vi "Read Flow Cal.vi"(8 "error in":errorcluster) -> (0 "error out":errorcluster, 2 "FM1-60":dbl[][](array[numeric]), 3 "FM1-20":dbl[][](array[numeric]))   [LabVIEW 2018]
uses:
  <vilib>/Utility/file.llb/Read Delimited Spreadsheet (DBL).vi
panel:
  # "GPM    HZ"
  # "GPM"
  # "HZ"
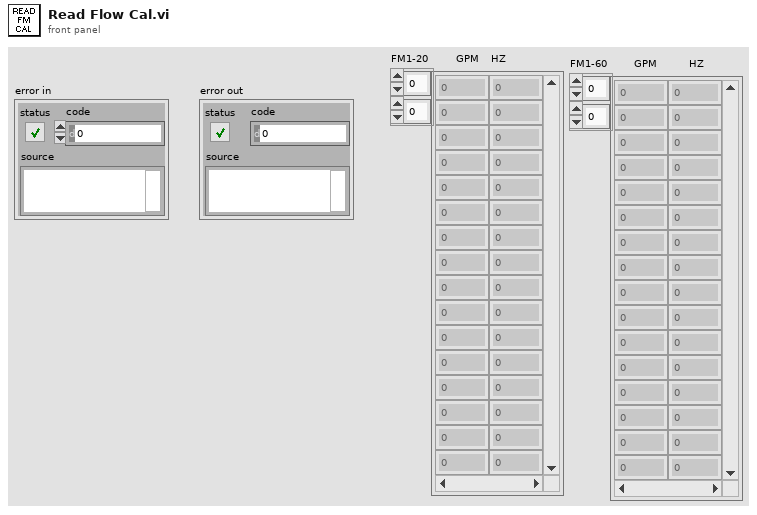
[diagram p1: front panel]
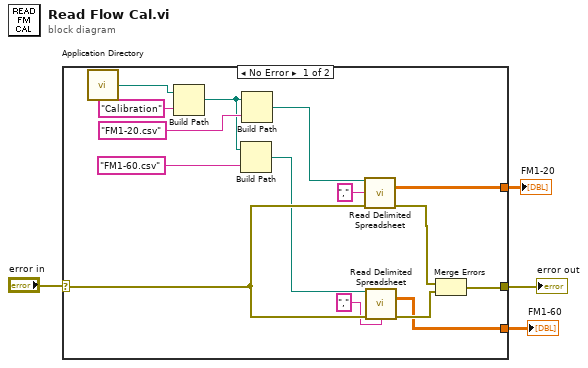
[diagram p0: block diagram]
diagram:
  n1 = case shown="No Error" "error in" {
    selector: "error in" -> [w19 w20]
    tunnel: [w12 w20] -> w3
    tunnel: [w6 _] -> w2
    tunnel: [w5 _] -> w1
    frame No Error {
      n2 = call <vilib>:"Application Directory.vi"() -> ("Application Directory"=w9:path)
      n3 = Build Path(base path=w9, name or relative path="Calibration") -> (appended path=w7:path)
      n4 = Build Path(base path=w7, name or relative path="FM1-60.csv") -> (appended path=w15:path)
      n5 = Build Path(base path=w7, name or relative path="FM1-20.csv") -> (appended path=w17:path)
      n6 = call-poly <vilib>:"Read Delimited Spreadsheet.vi"("file path (dialog if empty)"=w17, "error in (no error)"=w19, "delimiter (\\t)"="," ("delimiter (\\t)")) -> ("all rows"=w6:dbl[][], "error out"=w14:errorcluster)  [unwired: 7 in, 4 out]
      n7 = call-poly <vilib>:"Read Delimited Spreadsheet.vi"("file path (dialog if empty)"=w15, "error in (no error)"=w19, "delimiter (\\t)"="," ("delimiter (\\t)")) -> ("all rows"=w5:dbl[][], "error out"=w13:errorcluster)  [unwired: 7 in, 4 out]
      n8 = Merge Errors(w14, w13) -> (w12:errorcluster)
    }
    frame Error {
    }
  }
  "error out" <- w3
  "FM1-20" <- w2
  "FM1-60" <- w1
